vi "列表控件插入项符号.vi"() -> ()   [LabVIEW 2010]
uses:
  <vilib>/picture/picture.llb/imagedata.ctl
panel:
  in  "多列列表框":i32(listbox)
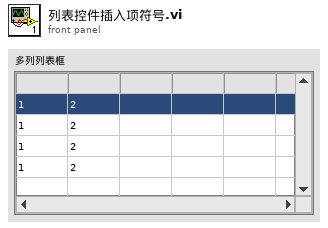
[diagram p1: front panel]
types:
  T1 = typedef "imagedata.ctl" = cluster{"image type":i32, "image depth":i32, "image":u8[], "mask":u8[], "colors":u32[], "Rectangle":cluster{"left":i16, "top":i16, "right":i16, "bottom":i16}}
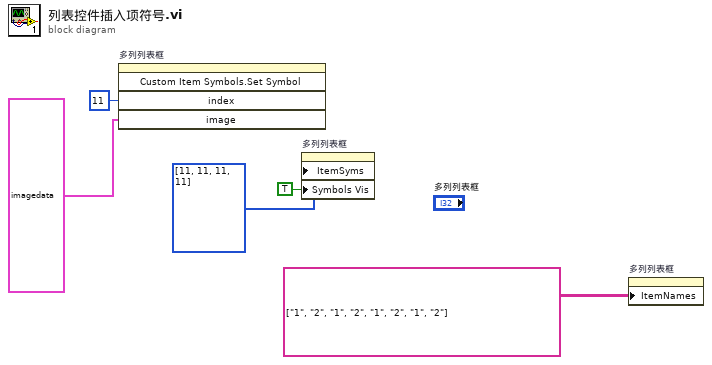
[diagram p0: block diagram]
diagram:
  n1 = invoke on="多列列表框" class="MCListbox (严格)" method="Custom Item Symbols.Set Symbol"("index"=11 ("索引"), "image"=T1 {"image type"=0, "image depth"=24, "image"=[255, 254, 255, 255, 254, 255, 255, 255, 253, 254, 255, 255, 255, 254, 253, 254, 255, 253, 254, 254, 254, 255, 255, 255, 254, 255, 255, 255, 254, 255, 254, 255, 253, 254, 255, 255, 255, 255, 255, 255, 255, 255, 255, 254, 255, 255, 255, 255, 255, 255, 251, 254, 255, 255, 255, 255, 253, 254, 255, 255, 255, 255, 255, 255, 255, 255, 255, 254, 255, 244, 255, 241, 220, 255, 223, 238, 255, 239, 255, 254, 255, 255, 254, 255, 255, 255, 253, 255, 255, 253, 254, 255, 255, 255, 254, 255, 255, 254, 255, 251, 255, 255, 255, 255, 255, 255, 255, 255, 254, 255, 255, 189, 254, 190, 117, 255, 116, 88, 255, 87, 78, 255, 76, 70, 255, 69, 83, 255, 84, 166, 255, 171, 255, 255, 253, 254, 254, 254, 255, 254, 255, 255, 255, 255, 255, 253, 254, 255, 254, 253, 255, 254, 251, 255, 255, 255, 150, 255, 150, 92, 254, 90, 88, 255, 89, 78, 255, 77, 71, 255, 71, 58, 254, 58, 45, 255, 44, 30, 255, 32, 110, 255, 111, 255, 254, 255, 255, 255, 255, 254, 255, 255, 255, 255, 255, 254, 255, 251, 255, 254, 255, 185, 255, 183, 85, 255, 88, 84, 255, 82, 73, 255, 75, 65, 255, 67, 52, 254, 54, 42, 255, 41, 30, 255, 29, 18, 255, 23, 7, 255, 9, 150, 255, 148, 255, 255, 255, 255, 254, 255, 255, 255, 255, 254, 255, 255, 254, 255, 255, 99, 254, 98, 80, 254, 77, 71, 255, 71, 63, 255, 60, 46, 255, 47, 35, 255, 35, 24, 255, 25, 13, 255, 13, 1, 255, 0, 5, 255, 0, 29, 255, 29, 254, 255, 253, 255, 255, 255, 255, 255, 255, 255, 254, 255, 219, 255, 219, 69, 255, 65, 61, 255, 63, 54, 255, 52, 38, 255, 38, 26, 255, 26, 13, 254, 15, 5, 255, 7, 0, 254, 0, 0, 254, 0, 1, 254, 3, 0, 255, 0, 213, 254, 214, 255, 254, 255, 254, 255, 255, 255, 255, 255, 200, 254, 202, 51, 254, 50, 44, 255, 45, 30, 255, 34, 23, 254, 24, 11, 255, 10, 3, 254, 0, 0, 255, 1, 0, 255, 0, 0, 255, 0, 0, 255, 1, 0, 255, 1, 184, 255, 185, 254, 255, 253, 255, 255, 255, 255, 254, 255, 211, 255, 215, 31, 255, 32, 25, 254, 29, 15, 254, 13, 5, 255, 5, 0, 255, 0, 0, 254, 0, 0, 255, 1, 0, 255, 1, 1, 255, 0, 0, 255, 1, 0, 255, 1, 207, 255, 207, 255, 255, 255, 255, 255, 253, 255, 255, 255, 250, 255, 252, 48, 254, 47, 8, 254, 5, 0, 255, 0, 0, 255, 1, 0, 253, 2, 1, 255, 0, 0, 255, 1, 0, 254, 0, 3, 254, 0, 0, 255, 3, 28, 255, 25, 255, 254, 255, 255, 255, 255, 254, 255, 255, 255, 255, 251, 255, 255, 253, 150, 255, 152, 1, 255, 1, 0, 255, 3, 0, 254, 0, 1, 254, 3, 0, 255, 3, 0, 255, 0, 1, 255, 0, 1, 255, 1, 0, 255, 0, 149, 254, 151, 255, 255, 253, 255, 255, 255, 254, 255, 255, 255, 255, 255, 255, 255, 255, 254, 255, 253, 93, 255, 92, 0, 255, 0, 3, 254, 0, 0, 255, 0, 1, 255, 0, 0, 255, 0, 1, 255, 1, 0, 255, 0, 95, 255, 95, 254, 255, 253, 250, 255, 255, 254, 255, 253, 255, 254, 255, 255, 254, 255, 255, 254, 255, 255, 254, 255, 255, 254, 255, 152, 254, 152, 33, 255, 30, 0, 255, 0, 0, 254, 0, 1, 255, 2, 28, 254, 32, 154, 255, 153, 255, 254, 255, 255, 254, 255, 255, 255, 255, 255, 254, 255, 253, 254, 255, 255, 254, 255, 255, 255, 255, 255, 255, 255, 252, 255, 255, 255, 254, 255, 253, 255, 254, 236, 255, 236, 205, 255, 204, 234, 255, 233, 255, 255, 253, 252, 255, 251, 255, 255, 255, 255, 253, 255, 255, 255, 255, 255, 255, 255, 255, 255, 255, 255, 255, 253, 251, 255, 255, 255, 255, 253, 255, 255, 255, 255, 254, 255, 255, 254, 255, 255, 254, 255, 255, 254, 255, 254, 254, 252, 255, 253, 255, 255, 255, 255, 255, 255, 253, 254, 254, 254, 255, 255, 255, 255, 255, 255, 254, 255, 253, 255, 255, 255, 255, 254, 255, 255, 255, 255, 254, 255, 253, 255, 255, 255, 254, 255, 255, 255, 255, 255, 253, 255, 254, 255, 255, 251, 255, 255, 255, 255, 255, 255, 255, 255, 253, 255, 254, 255, 255, 254, 252, 254, 255, 255], "mask"=[], "colors"=[], "Rectangle"={"left"=0, "top"=0, "right"=16, "bottom"=16}} ("image data")) -> ()  [unwired: 3 in, 5 out]
  n2 = property on="多列列表框" class="MCListbox (严格)"("ItemSyms"=i32[] [11, 11, 11, 11] ("项符号"), "Symbols Vis"=TRUE ("显示项:显示符号")) -> ()  [unwired: 2 in, 2 out]
  n3 = property on="多列列表框" class="MCListbox (严格)"("ItemNames"=string[][] [["1", "2"], ["1", "2"], ["1", "2"], ["1", "2"]] ("项名")) -> ()  [unwired: 2 in, 2 out]
